vi "Read ESPAÑOL.vi"(8 "error in (no error)":errorcluster, 11 "CAFE ACTOR in":refnum<class "CAFE ACTOR.lvclass">) -> (0 "error out":errorcluster, 2 "ESPAÑOL":bool, 3 "CAFE ACTOR out":refnum<class "CAFE ACTOR.lvclass">)   [LabVIEW 2019, in "CAFE ACTOR.lvlib" / "CAFE ACTOR.lvclass"]
uses:
  CAFE ACTOR.lvclass
  CAFE ACTOR.lvclass/CAFE ACTOR.ctl
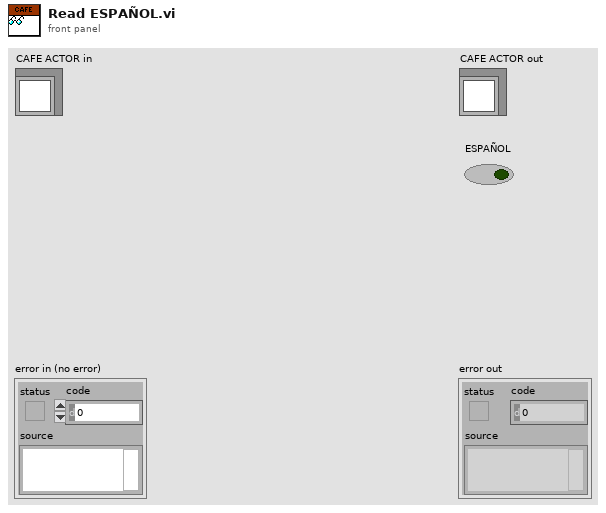
[diagram p1: front panel]
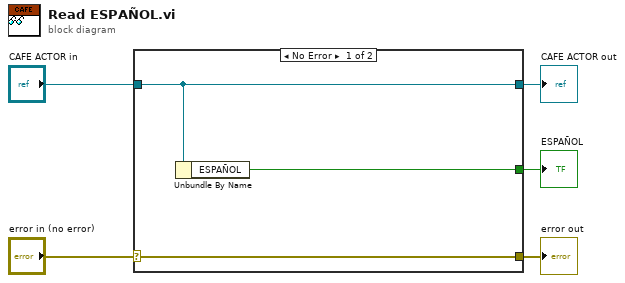
[diagram p0: block diagram]
diagram:
  n1 = case shown="No Error" "error in (no error)" {
    selector: "error in (no error)" -> [w8 w9]
    tunnel: [w8 w9] -> w4
    tunnel: [w7 w10] -> w2
    tunnel: "CAFE ACTOR in" -> [w7 w10]
    tunnel: [w6 _] -> w1
    frame No Error {
      n2 = Unbundle By Name(w7) -> ("ESPAÑOL"=w6:bool)
    }
    frame Error {
    }
  }
  "error out" <- w4
  "CAFE ACTOR out" <- w2
  "ESPAÑOL" <- w1
